vi "saveCleanly.vi"(6 "Node Refnum CDS New":refnum<vi>, 8 "error in (no error)":errorcluster, 9 "Block Diagram":refnum<vi>, 10 "vi reference":refnum<vi>, 11 "VI in":refnum<class "VI.lvclass">) -> (0 "error out":errorcluster, 3 "VI out":refnum<class "VI.lvclass">)   [LabVIEW 2016, in "VI.lvclass"]
uses:
  VI.lvclass
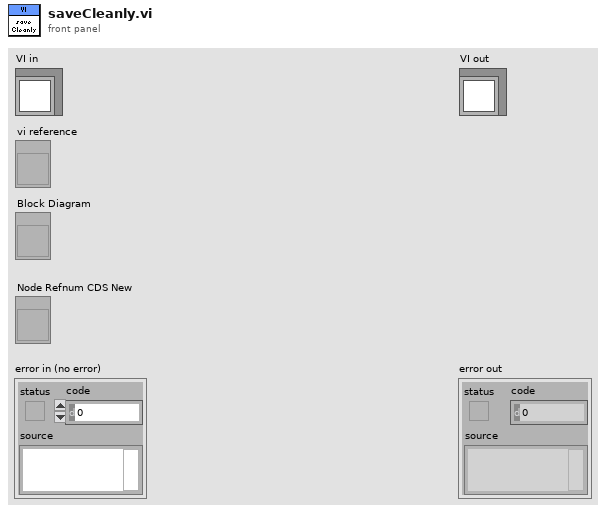
[diagram p1: front panel]
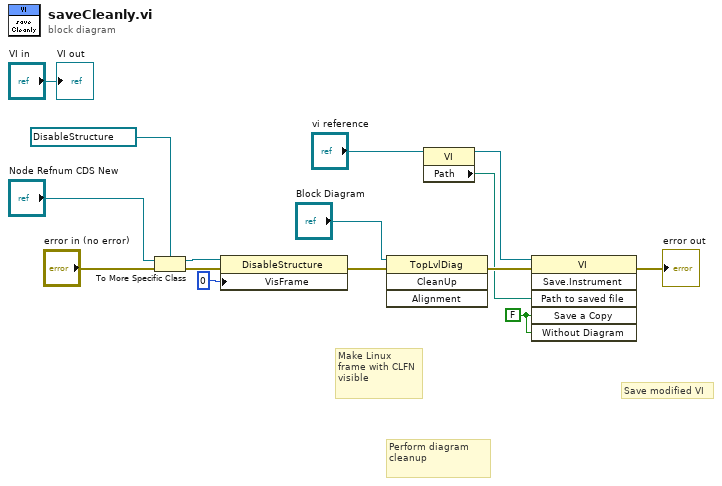
[diagram p0: block diagram]
diagram:
  w11 = FALSE ("Save a Copy")
  # "Save modified VI"
  # "Perform diagram cleanup"
  # "Make Linux frame with CLFN visible"
  n1 = To More Specific Class(target class=refnum<vi> refnum ("EnclosureType"), reference="Node Refnum CDS New", error in="error in (no error)") -> (specific class reference=w4:refnum<vi>, error out=w2:errorcluster)
  n2 = property class="DisableStructure"(reference=w4, error in=w2, "VisFrame"=u32 0 ("Visible Frame")) -> (error out=w13:errorcluster)  [unwired: 1 out]
  n3 = invoke class="TopLvlDiag" method="CleanUp"(reference="Block Diagram", error in=w13) -> (error out=w12:errorcluster)  [unwired: 2 in, 3 out]
  n4 = property on="Property Node" class="VI"(reference="vi reference") -> (reference out=w7:refnum<vi>, "Path"=w8:path)  [unwired: 1 in, 1 out]
  n5 = invoke class="VI" method="Save.Instrument"(reference=w7, error in=w12, "Path to saved file"=w8, "Save a Copy"=w11, "Without Diagram"=w11) -> (error out=→"error out":errorcluster)  [unwired: 1 in, 5 out]
  "VI out" <- "VI in"
